vi "sslSimulationProtocolRobotControlResponse.vi"(8 "error in (no error)":errorcluster, 11 "robotControlArray":u8[](array[numeric])) -> (0 "error out":errorcluster, 3 "RobotsFeedback":refnum<class "RobotFeedback.lvclass">[](array[class]))   [LabVIEW 2023, in "Communication.lvclass"]
uses:
  Communication.lvclass
  RobotFeedback/RobotFeedback.lvclass
panel:
  out "Communication out":refnum<class "Communication.lvclass">
  in  "Communication in":refnum<class "Communication.lvclass">
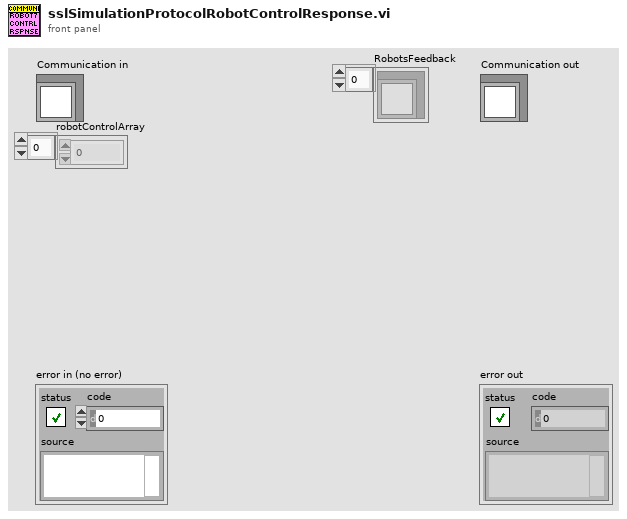
[diagram p1: front panel]
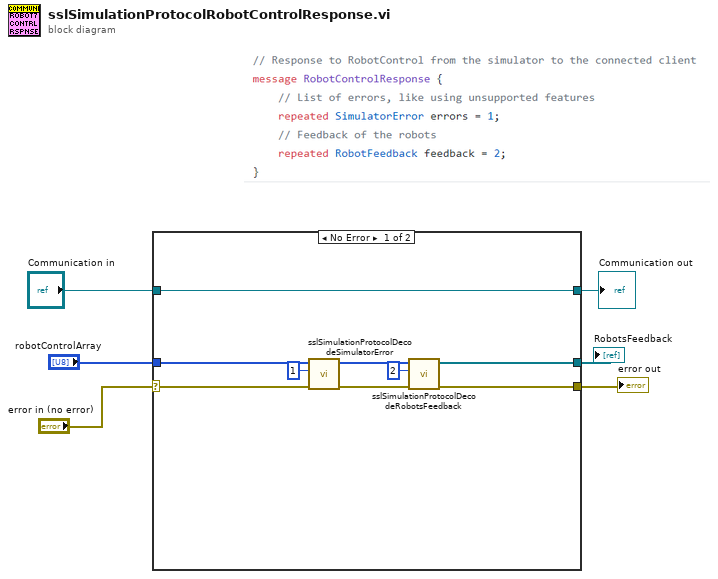
[diagram p0: block diagram]
diagram:
  n1 = case shown="No Error" "error in (no error)" {
    selector: "error in (no error)" -> [w10 w17]
    tunnel: [w8 w17] -> w5
    tunnel: [w15 w16] -> w3
    tunnel: "Communication in" -> [w15 w16]
    tunnel: "robotControlArray" -> [w14 _]
    tunnel: [w7 _] -> w1
    frame No Error {
      n2 = call "sslSimulationProtocolDecodeSimulatorError.vi"("error in"=w10, "Key"=1, "robotControlResponseArray"=w14) -> ("error out"=w9:errorcluster, "array w/ subset deleted"=w13:u8[])  [unwired: 7 in]
      n3 = call "sslSimulationProtocolDecodeRobotsFeedback.vi"("error in (no error)"=w9, "Key"=2, "robotsFeedbackArray"=w13) -> ("error out"=w8:errorcluster, "RobotsFeedback"=w7:refnum<class "RobotFeedback.lvclass">[])  [unwired: 7 in]
    }
    frame Error {
    }
  }
  "error out" <- w5
  "Communication out" <- w3
  "RobotsFeedback" <- w1
